vi "Data_Balancing.vi"(11 "Array in":sgl[][](array[numeric])) -> (3 "Array out":sgl[][](array[numeric]))   [LabVIEW 2020]
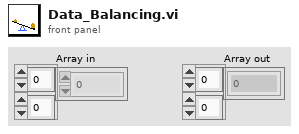
[diagram p1: front panel]
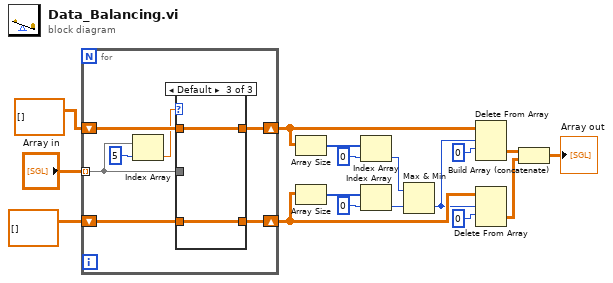
[diagram p0: block diagram]
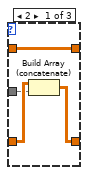
[diagram p2: hidden frame]
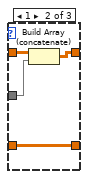
[diagram p3: hidden frame]
diagram:
  n1 = for {
    tunnel: "Array in" -> [w20] mode=indexing
    shift-right: [w19] -> w13
    shift-left: sgl[][] [] -> [w23]
    shift-right: [w18] -> w10
    shift-left: sgl[][] [] -> [w22]
    n2 = Index Array(array=w20, index=5) -> (element=w21:sgl)
    n3 = case shown="Default" w21 {
      tunnel: w23 -> [w28 w29 w33]
      tunnel: w22 -> [w25 w32 w34]
      tunnel: w20 -> [w27 w31 _]
      tunnel: [w26 w29 w33] -> w19
      tunnel: [w25 w30 w34] -> w18
      frame 2 {
        n4 = Build Array (concatenate)(w28, w27) -> (w26:sgl[][])
      }
      frame 1 {
        n5 = Build Array (concatenate)(w32, w31) -> (w30:sgl[][])
      }
      frame Default {
      }
    }
  }
  n6 = Array Size(array=w10) -> (size(s)=w4:i32[])
  n7 = Array Size(array=w13) -> (size(s)=w7:i32[])
  n8 = Index Array(array=w4, index=0) -> (element=w8:i32)
  n9 = Index Array(array=w7, index=0) -> (element=w9:i32)
  n10 = Max & Min(x=w8, y=w9) -> (min(x,y)=w12:i32)  [unwired: 1 out]
  n11 = Delete From Array(array=w10, length=w12, index (row)=0) -> (deleted portion=w16:sgl[][])  [unwired: 1 in, 1 out]
  n12 = Delete From Array(array=w13, length=w12, index (row)=0) -> (deleted portion=w17:sgl[][])  [unwired: 1 in, 1 out]
  n13 = Build Array (concatenate)(w16, w17) -> (→"Array out":sgl[][])
